vi "reset_io_to_default.vi"(8 "error in (no error)":errorcluster, 11 "Modbus Master in":refnum<class "Modbus Master.lvclass">) -> (0 "error out":errorcluster, 3 "Modbus Master out":refnum<class "Modbus Master.lvclass">)   [LabVIEW 2018, in "ICP xET-7017.lvlib"]
uses:
  ICP xET-7017.lvlib
  <vilib>/NI/Modbus Library/API/Master/Modbus Master.lvclass
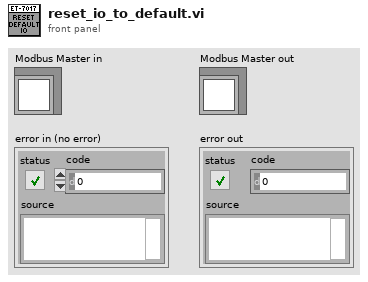
[diagram p1: front panel]
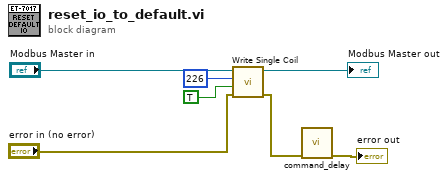
[diagram p0: block diagram]
diagram:
  n1 = call-dynamic "Write Single Coil.vi"("error in"="error in (no error)", "coil to write"=TRUE, "address"=u16 226 ("starting address"), "Modbus master in"="Modbus Master in") -> ("error out"=w2:errorcluster, "Modbus master out"=→"Modbus Master out":refnum<class "Modbus Master.lvclass">)  [unwired: 6 in]
  n2 = call "command_delay.vi"("error in (no error)"=w2) -> ("error out"=→"error out":errorcluster)  [unwired: 10 in]
